vi "Citroen c4.vi"() -> ()   [LabVIEW 2021, in "uCanDriver.lvlib" / "uCAN.lvclass"]
uses:
  uCAN.lvclass
  typedefs/bitrates.ctl
  typedefs/frame.ctl
  typedefs/control leds.ctl
panel:
  in  "speed limit":i16
  in  "Cruise type":enum16{"Off", "On cruise", "On limit"}(ring)
  in  "out of gas warning":bool
  in  "Trip":dbl
  in  "Slide":u8(slide) scale=0.0..12.0
  in  "Gear":T1(ring)
  in  "Cluster":T2
  in  "Ignition":bool
  in  "Odometer":i32
  in  "Speed":u16(slide) scale=0.0..250.0
  in  "Disable markers":bool
  in  "Panel Backlight":u8(slide) max=15 step=1 scale=0.0..15.0
  out "Array":T3[](array[typedef]) {"Data" format="%.0x"; "ID" format="%.0x"}
  in  "Bitrates":T4=enum."500 kbit/s"
  in  "COM port":refnum<visa-resource-name>="COM9"
  in  "stop":bool
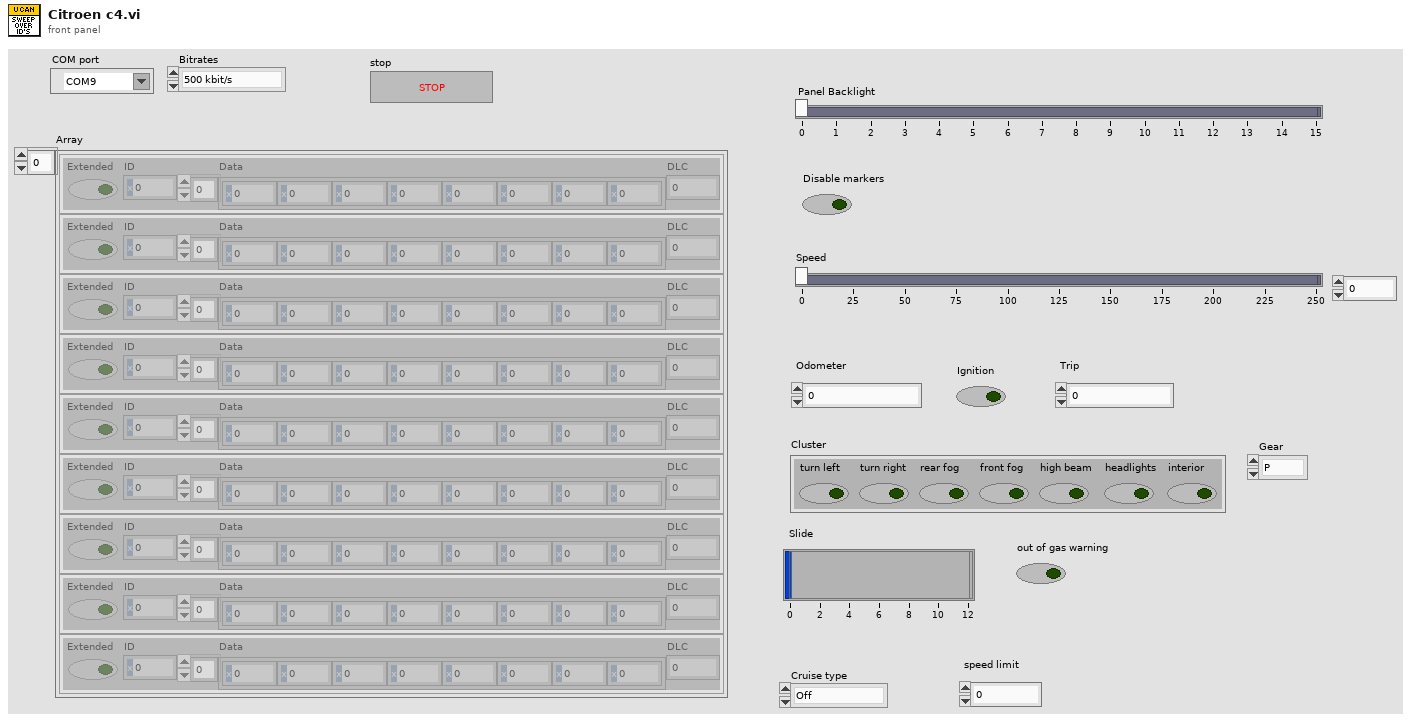
[diagram p1: front panel]
types:
  T1 = enum16{"P", "R", "N", "-", "6", "5", "4", "3", "2", "1", ""}
  T2 = typedef "control leds.ctl" = cluster{"turn left":bool, "turn right":bool, "rear fog":bool, "front fog":bool, "high beam":bool, "headlights":bool, "interior":bool}
  T3 = typedef "uCanDriver.lvlib/uCAN.lvclass/frame.ctl" = cluster{"Extended":bool, "ID":u32, "Data":u8[], "DLC":u8}
  T4 = typedef "uCanDriver.lvlib/uCAN.lvclass/bitrates.ctl" = enum16{"100 kbit/s", "125 kbit/s", "250 kbit/s", "500 kbit/s", "800 kbit/s", "1 Mbit/s"}
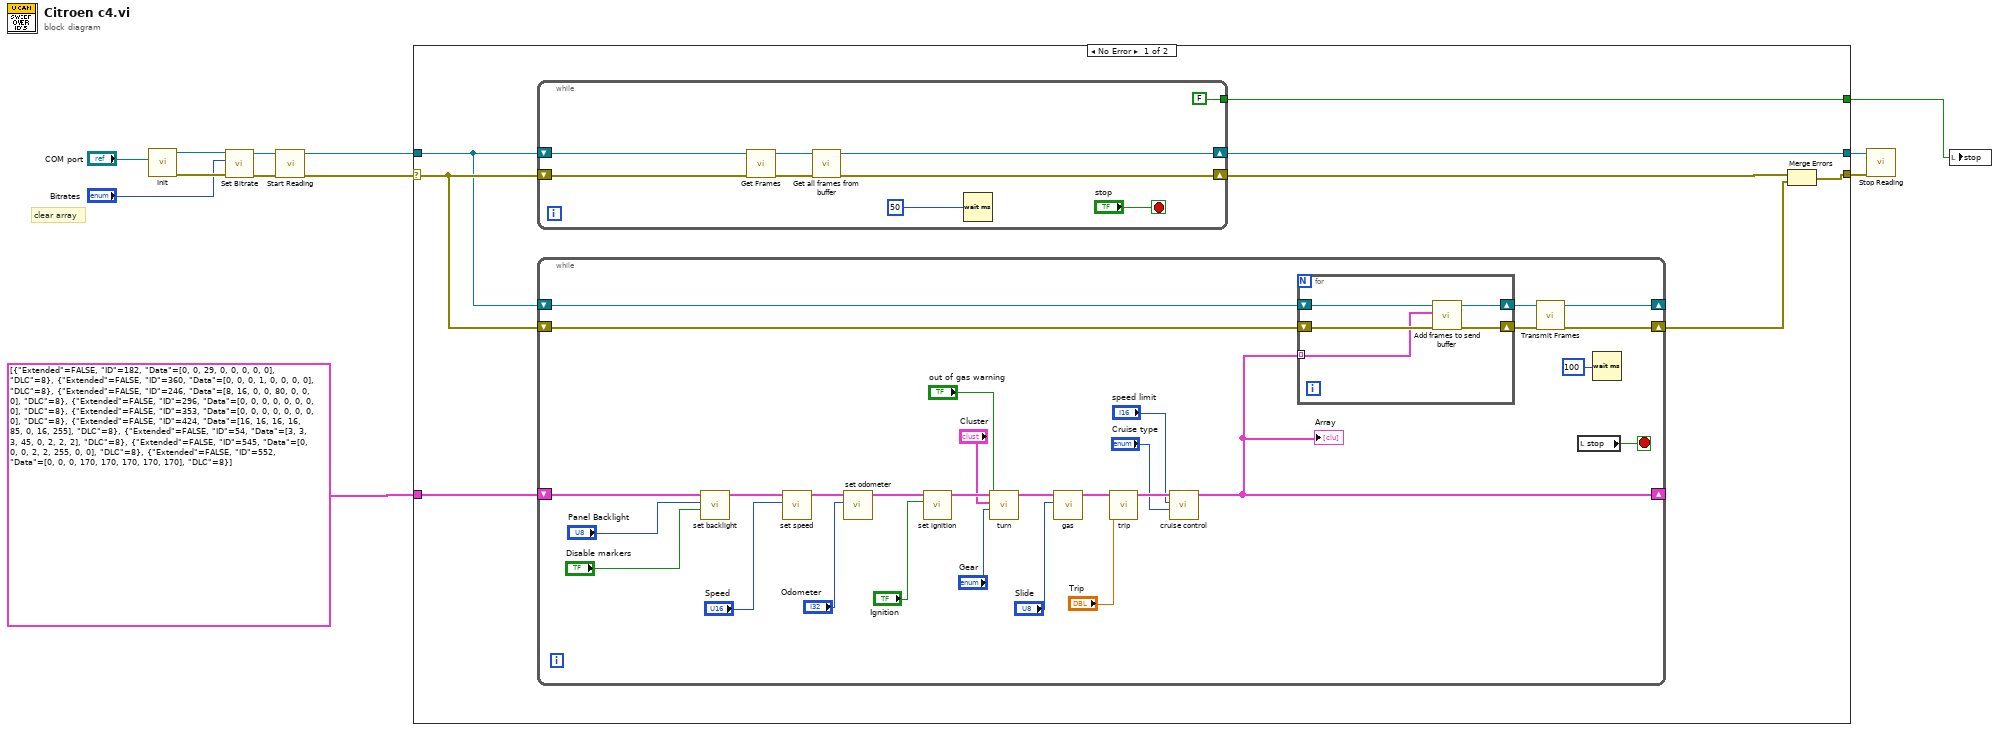
[diagram p0: block diagram]
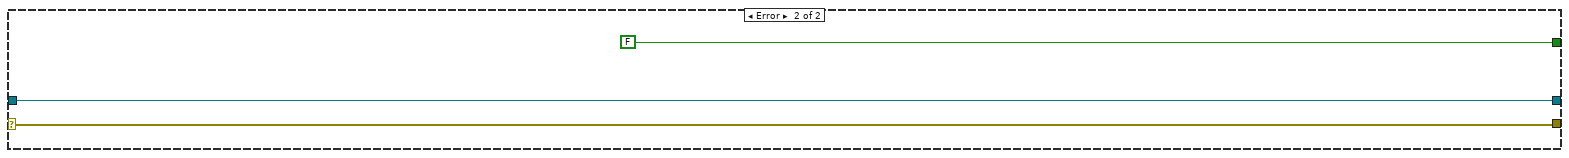
[diagram p2: hidden frame]
diagram:
  # "clear array"
  n1 = call "Init.vi"("COM port"="COM port") -> ("error out"=w10:errorcluster, "uCAN out"=w11:refnum<class "uCAN.lvclass">)  [unwired: 9 in]
  n2 = call "Set Bitrate.vi"("error in (no error)"=w10, "Bitrates"="Bitrates", "uCAN in"=w11) -> ("error out"=w6:errorcluster, "uCAN out"=w4:refnum<class "uCAN.lvclass">)  [unwired: 7 in]
  n3 = call "Start Reading.vi"("error in (no error)"=w6, "uCAN in"=w4) -> ("error out"=w5:errorcluster, "uCAN out"=w3:refnum<class "uCAN.lvclass">)  [unwired: 8 in]
  n4 = case shown="No Error" w5 {
    selector: w5 -> [w16 w66]
    tunnel: [w20 w65] -> w8
    tunnel: [w18 w66] -> w7
    tunnel: w3 -> [w15 w65]
    tunnel: [w14 FALSE ("stop")] -> w2
    tunnel: T3[] [{"Extended"=FALSE, "ID"=182, "Data"=[0, 0, 29, 0, 0, 0, 0, 0], "DLC"=8}, {"Extended"=FALSE, "ID"=360, "Data"=[0, 0, 0, 1, 0, 0, 0, 0], "DLC"=8}, {"Extended"=FALSE, "ID"=246, "Data"=[8, 16, 0, 0, 80, 0, 0, 0], "DLC"=8}, {"Extended"=FALSE, "ID"=296, "Data"=[0, 0, 0, 0, 0, 0, 0, 0], "DLC"=8}, {"Extended"=FALSE, "ID"=353, "Data"=[0, 0, 0, 0, 0, 0, 0, 0], "DLC"=8}, {"Extended"=FALSE, "ID"=424, "Data"=[16, 16, 16, 16, 85, 0, 16, 255], "DLC"=8}, {"Extended"=FALSE, "ID"=54, "Data"=[3, 3, 3, 45, 0, 2, 2, 2], "DLC"=8}, {"Extended"=FALSE, "ID"=545, "Data"=[0, 0, 0, 2, 2, 255, 0, 0], "DLC"=8}, {"Extended"=FALSE, "ID"=552, "Data"=[0, 0, 0, 170, 170, 170, 170, 170], "DLC"=8}] ("Array") -> [w13 _]
    frame No Error {
      n5 = while {
        shift-right: [w59] -> w20
        shift-left: w15 -> [w63]
        shift-right: [w58] -> w19
        shift-left: w16 -> [w62]
        tunnel: [FALSE ("stop")] -> w14
        stop <- "stop" stop-if-true
        n6 = call "Get Frames.vi"("error in (no error)"=w62, "uCAN in"=w63) -> ("error out"=w61:errorcluster, "uCAN out"=w60:refnum<class "uCAN.lvclass">)  [unwired: 7 in, 1 out]
        n7 = call "Get all frames from buffer.vi"("error in (no error)"=w61, "uCAN in"=w60) -> ("error out"=w58:errorcluster, "uCAN out"=w59:refnum<class "uCAN.lvclass">)  [unwired: 7 in, 1 out]
        n8 = Wait (ms)(milliseconds to wait=u32 50) -> ()  [unwired: 1 out]
      }
      n9 = while {
        shift-right: [w44] -> _
        shift-left: w15 -> [w49]
        shift-right: [w46] -> w17
        shift-left: w16 -> [w48]
        shift-right: [w23] -> _
        shift-left: w13 -> [w41]
        stop <- w43 stop-if-true
        n10 = call "set backlight.vi"("Disable markers"="Disable markers", "Panel Backlight"="Panel Backlight", "Array"=w41) -> ("Array 2"=w38:T3[])  [unwired: 8 in]
        n11 = call "set speed.vi"("Speed"="Speed", "Array"=w38) -> ("Array 2"=w36:T3[])  [unwired: 9 in]
        n12 = call "set odometer.vi"("Odometer"="Odometer", "Array"=w36) -> ("Array 2"=w34:T3[])  [unwired: 9 in]
        n13 = call "set ignition.vi"("Ignition"="Ignition", "Array"=w34) -> ("Array 2"=w32:T3[])  [unwired: 9 in]
        n14 = call "turn.vi"("out of gas warning"="out of gas warning", "Gear"="Gear", "Cluster"="Cluster", "Array"=w32) -> ("Array 2"=w29:T3[])  [unwired: 7 in]
        n15 = call "gas.vi"("Slide"="Slide", "Array"=w29) -> ("Array 2"=w27:T3[])  [unwired: 9 in]
        n16 = call "trip.vi"("Trip"="Trip", "Array"=w27) -> ("Array 2"=w24:T3[])  [unwired: 9 in]
        n17 = call "cruise control.vi"("Cruise type"="Cruise type", "speed limit"="speed limit", "Array"=w24) -> ("Array 2"=w23:T3[])  [unwired: 8 in]
        "Array" <- w23
        n18 = for {
          shift-right: [w51] -> w45
          shift-left: w49 -> [w54]
          shift-right: [w52] -> w47
          shift-left: w48 -> [w53]
          tunnel: w23 -> [w50] mode=indexing
          n19 = call "Add frames to send buffer.vi"("error in (no error)"=w53, "New Frame"=w50, "uCAN in"=w54) -> ("error out"=w52:errorcluster, "uCAN out"=w51:refnum<class "uCAN.lvclass">)  [unwired: 7 in]
        }
        n20 = call "Transmit Frames.vi"("error in (no error)"=w47, "uCAN in"=w45) -> ("error out"=w46:errorcluster, "uCAN out"=w44:refnum<class "uCAN.lvclass">)  [unwired: 8 in]
        n21 = local read "stop"() -> (w43:bool)
        n22 = Wait (ms)(milliseconds to wait=u32 100) -> ()  [unwired: 1 out]
      }
      n23 = Merge Errors(w19, w17) -> (w18:errorcluster)
    }
    frame Error {
    }
  }
  n24 = call "Stop Reading.vi"("error in (no error)"=w7, "uCAN in"=w8) -> ()  [unwired: 8 in, 2 out]
  n25 = local write "stop"(w2) -> ()
